vi "Configure Adjacent Channel Power (In Band Setup).vi"(0 "VISA resource name":refnum<visa-resource-name>, 1 "ACP Filter Target Type (0:Both)":i32(ring) items=["Both", "In Band", "Offset Channel"], 2 "ACP Filter (1:Nyquist)":i32(ring)=1 items=["Rectangular", "Nyquist", "Root Nyquist"], 3 "ACP Ratio Target  (0:In Band)":i32(ring) items=["In Band", "Offset Channel"], 5 "ACP Carrier Number (1)":i32=1 min=1 max=12, 7 "ACP Frequency (1325000000Hz)":dbl=1325000000.0, 9 "ACP Bandwidth (3840000Hz)":dbl=3840000.0 min=1.0 max=1000000000.0, 11 "error in (no error)":errorcluster, 12 "ACP Interval (5000000Hz)":dbl=5000000.0 min=0.0 max=1000000000.0, 13 "ACP Ratio (0.22)":dbl=0.22 min=0.01 max=1.0 format="%.2f") -> (4 "VISA resource name out":refnum<visa-resource-name>, 15 "error out":errorcluster)   [LabVIEW 2020, in "Anritsu Signal Analyzer Series.lvlib"]
doc: "Configures the in band for ACP measurement of the spectrum analyzer."
uses:
  Anritsu Signal Analyzer Series.lvlib
panel:
  # "Hz"
  # "Hz"
  # "Hz"
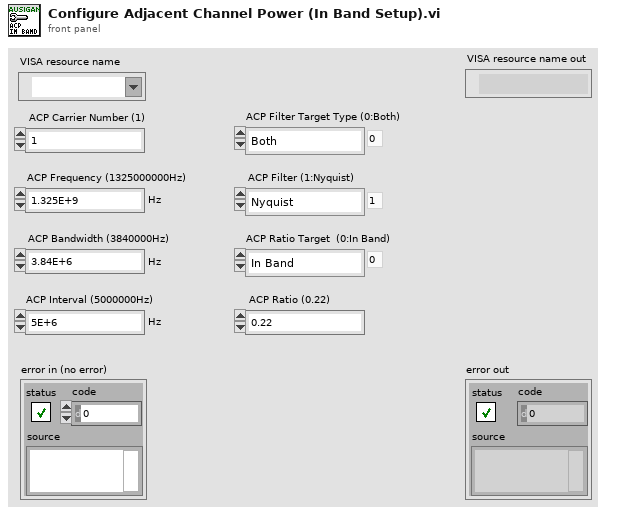
[diagram p1: front panel]
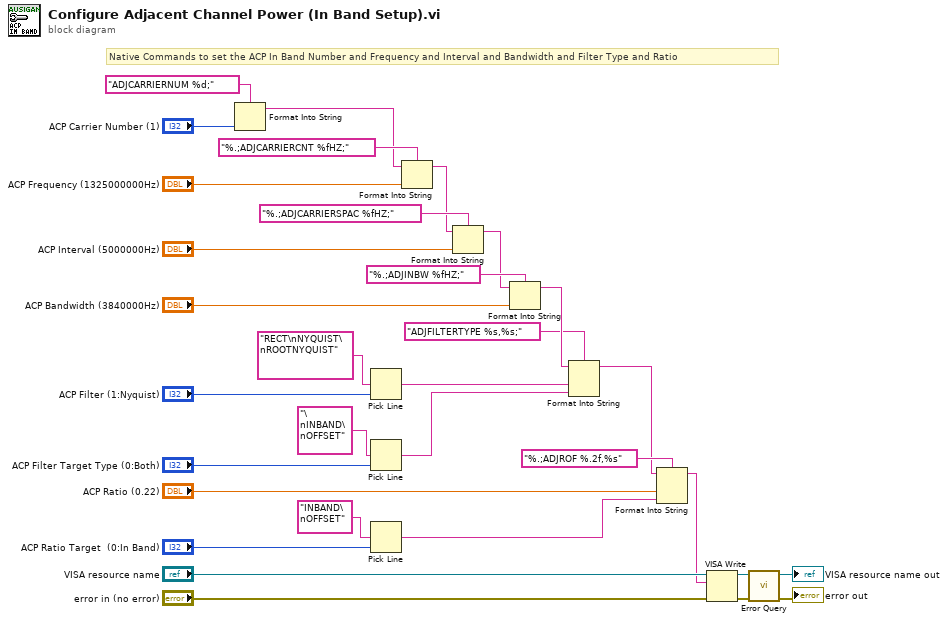
[diagram p0: block diagram]
diagram:
  # "Native Commands to set the ACP In Band Number and Frequency and Interval and Bandwidth and Filter Type and Ratio"
  n1 = Format Into String(format string="ADJCARRIERNUM %d;" ("Format String"), "ACP Carrier Number (1)") -> (resulting string=w18:string)  [unwired: 2 in, 1 out]
  n2 = Pick Line(multi-line string="RECT\nNYQUIST\nROOTNYQUIST" ("複数行文字列"), line index="ACP Filter (1:Nyquist)") -> (output string=w4:string)  [unwired: 1 in]
  n3 = Pick Line(multi-line string="\nINBAND\nOFFSET" ("複数行文字列"), line index="ACP Filter Target Type (0:Both)") -> (output string=w1:string)  [unwired: 1 in]
  n4 = Pick Line(multi-line string="INBAND\nOFFSET" ("複数行文字列"), line index="ACP Ratio Target  (0:In Band)") -> (output string=w3:string)  [unwired: 1 in]
  n5 = Format Into String(format string="%.;ADJCARRIERCNT %fHZ;" ("Format String"), initial string=w18, "ACP Frequency (1325000000Hz)") -> (resulting string=w16:string)  [unwired: 1 in, 1 out]
  n6 = Format Into String(format string="%.;ADJCARRIERSPAC %fHZ;" ("Format String"), initial string=w16, "ACP Interval (5000000Hz)") -> (resulting string=w14:string)  [unwired: 1 in, 1 out]
  n7 = Format Into String(format string="%.;ADJINBW %fHZ;" ("Format String"), initial string=w14, "ACP Bandwidth (3840000Hz)") -> (resulting string=w13:string)  [unwired: 1 in, 1 out]
  n8 = Format Into String(format string="ADJFILTERTYPE %s,%s;" ("_CommandSet"), initial string=w13, w4, w1) -> (resulting string=w10:string)  [unwired: 1 in, 1 out]
  n9 = Format Into String(format string="%.;ADJROF %.2f,%s" ("Format String"), initial string=w10, "ACP Ratio (0.22)", w3) -> (resulting string=w7:string)  [unwired: 1 in, 1 out]
  n10 = VISA Write(VISA resource name="VISA resource name", write buffer=w7, error in (no error)="error in (no error)") -> (VISA resource name out=w9:refnum<visa-resource-name>, error out=w8:errorcluster)  [unwired: 1 out]
  n11 = call "Error Query.vi"("error in (no error)"=w8, "VISA resource name"=w9) -> ("error out"=→"error out":errorcluster, "VISA resource name out"=→"VISA resource name out":refnum<visa-resource-name>)  [unwired: 6 in, 2 out]
